vi "numberpad.vi"() -> (3 "String":string)   [LabVIEW 2014, in "Master.lvclass"]
uses:
  Master/Master.lvclass
panel:
  in  "Tab Control":enum32{"Page 1", "Page 2"}(tab)
  in  "Enter":bool
  in  ".":bool
  in  "1":bool
  in  "2":bool
  in  "3":bool
  in  "4":bool
  in  "5":bool
  in  "6":bool
  in  "7":bool
  in  "8":bool
  in  "9":bool
  in  "0":bool
  in  "DEL":bool
  in  "String (in)":string
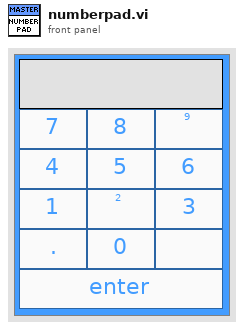
[diagram p1: front panel]
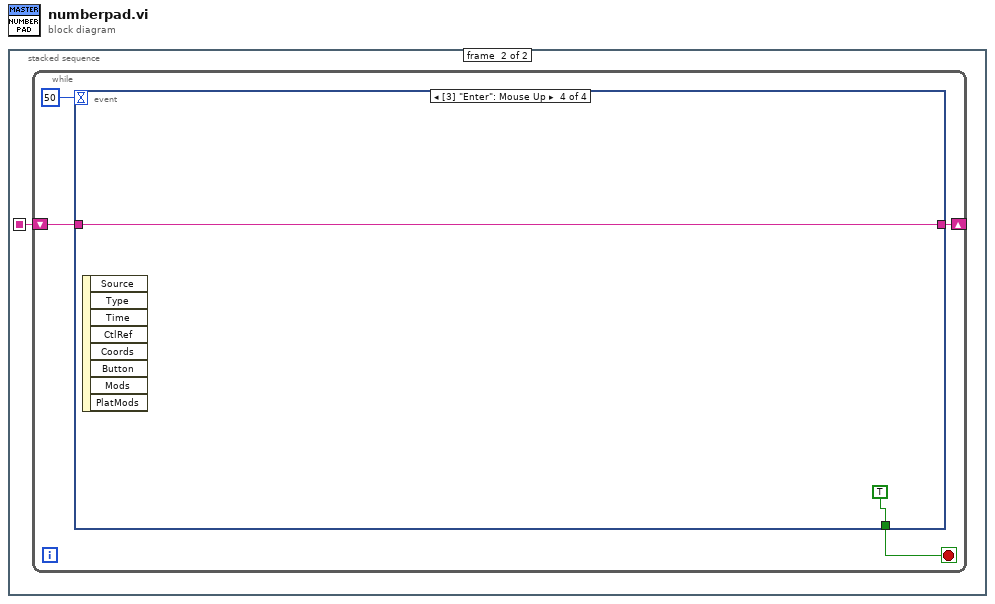
[diagram p0: block diagram]
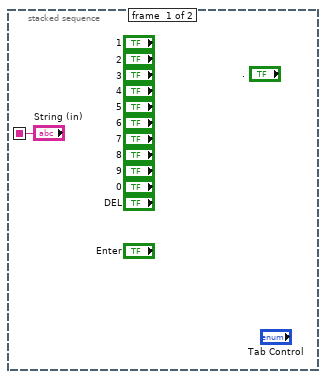
[diagram p2: hidden frame]
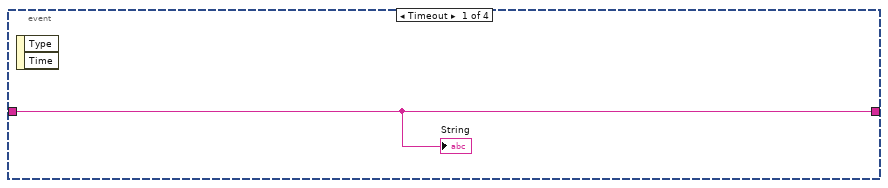
[diagram p3: hidden frame]
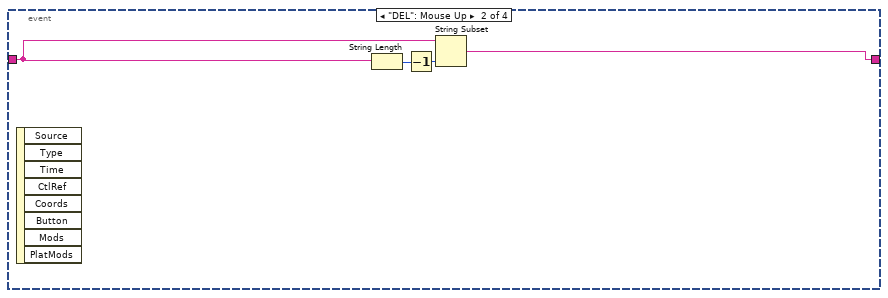
[diagram p4: hidden frame]
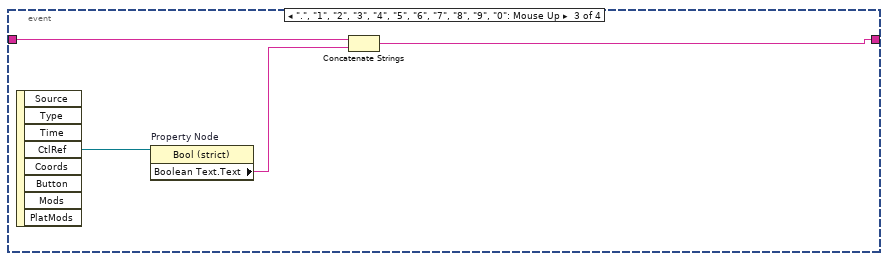
[diagram p5: hidden frame]
diagram:
  n1 = stacked-sequence {
    seq-local: ["String (in)" _] -> [_ w2]
    frame #0 {
    }
    frame #1 {
      n2 = while {
        shift-right: [w5] -> _
        shift-left: w2 -> [w6]
        stop <- w4 stop-if-true
        n3 = event shown="[3] \"Enter\": Mouse Up" {
          selector: _ -> [_ _ _ _]
          dyn-events: _ -> [_ _ _ _]
          timeout: 50 -> [_ _ _ _]
          tunnel: w6 -> [w7 w11 w15 w16]
          tunnel: [w7 w8 w14 w16] -> w5
          tunnel: [_ _ _ TRUE] -> w4
          event Timeout {
            n4 = event-data() -> ()  [unwired: 1 in, 2 out]
            "String" <- w7
          }
          event "DEL": Mouse Up {
            n5 = event-data() -> ()  [unwired: 1 in, 8 out]
            n6 = String Length(string=w11) -> (length=w10:i32)
            n7 = Decrement(x=w10) -> (x-1=w9:i32)
            n8 = String Subset(string=w11, length (rest)=w9) -> (substring=w8:string)  [unwired: 1 in]
          }
          event ".", "1", "2", "3", "4", "5", "6", "7", "8", "9", "0": Mouse Up {
            n9 = event-data() -> ("CtlRef"=w13:refnum<vi>)  [unwired: 1 in, 7 out]
            n10 = property on="Property Node" class="Bool (strict)"(reference=w13) -> ("Boolean Text.Text"=w12:string)  [unwired: 1 in, 2 out]
            n11 = Concatenate Strings "Concatenate Strings"(w15, w12) -> (w14:string)
          }
          event "Enter": Mouse Up {
            n12 = event-data() -> ()  [unwired: 1 in, 8 out]
          }
        }
      }
    }
  }
